vi "Pause.vi"(8 "error in (no error)":errorcluster, 11 "SS P100 Settings In":T1) -> (0 "error out":errorcluster, 1 "Connection Error":bool, 3 "SS P100 Settings Out":T1)   [LabVIEW 2018, in "Sonic Systems P100.lvlib"]
uses:
  Sonic Systems P100.lvlib
  Sonic Systems P100 Settings.ctl
  support/Support Library.lvlib
panel:
  out "read buffer":string
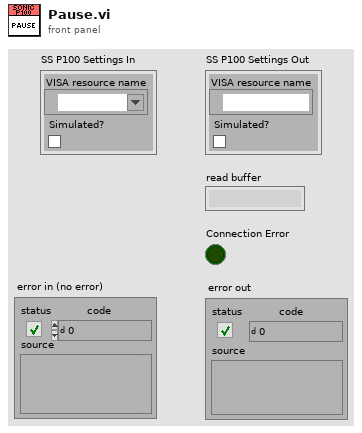
[diagram p1: front panel]
types:
  T1 = typedef "Sonic Systems P100.lvlib/Sonic Systems P100 Settings.ctl" = cluster{"VISA resource name":refnum<visa-resource-name>, "Simulated?":bool}
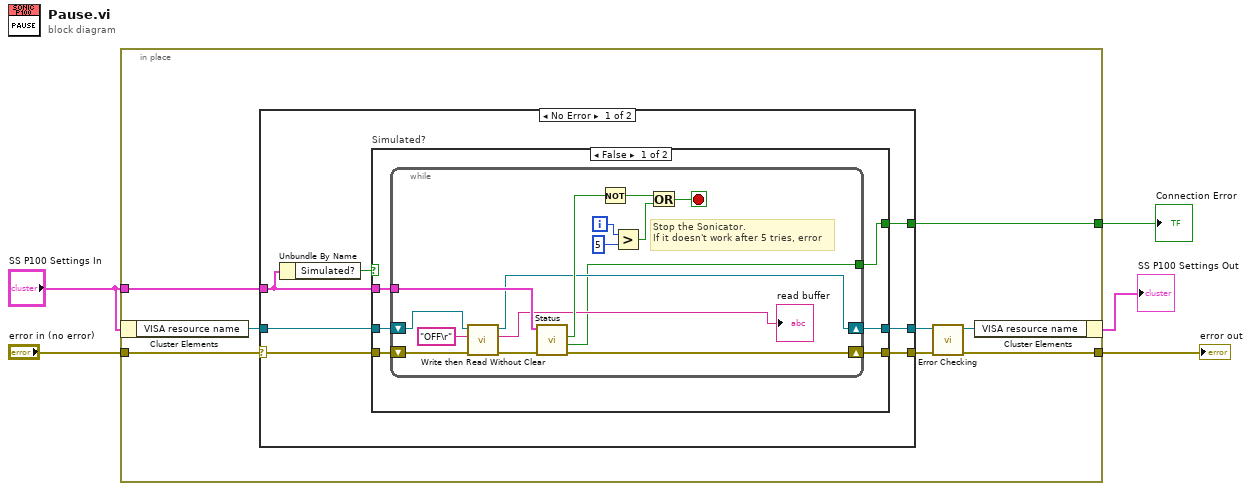
[diagram p0: block diagram]
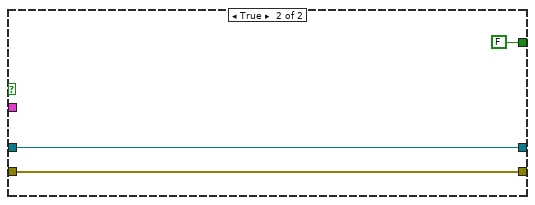
[diagram p2: hidden frame]
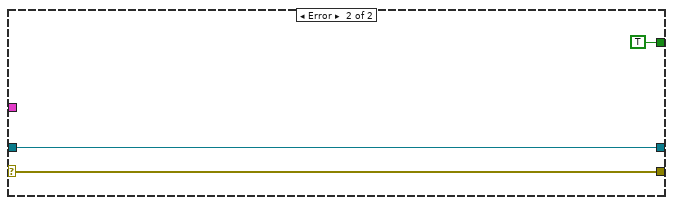
[diagram p3: hidden frame]
diagram:
  n1 = in-place {
    in-place-border: "error in (no error)" -> [w13]
    in-place-border: [w10] -> w4
    in-place-border: "SS P100 Settings In" -> [w9]
    in-place-border: [w6] -> w1
    n2 = in-place-cluster #1("SS P100 Settings In") -> ("VISA resource name"=w8:refnum<visa-resource-name>)
    n3 = case shown="No Error" w13 {
      selector: w13 -> [w20 w47]
      tunnel: w9 -> [w16 _]
      tunnel: [w19 w47] -> w11
      tunnel: [w18 w46] -> w12
      tunnel: w8 -> [w15 w46]
      tunnel: [w14 TRUE ("Connection Error")] -> w6
      frame No Error {
        n4 = Unbundle By Name(w16) -> ("Simulated?"=w17:bool)
        n5 = case "Simulated?" shown="False" w17 {
          tunnel: w20 -> [w24 w44]
          tunnel: [w22 w44] -> w19
          tunnel: [w26 w43] -> w18
          tunnel: w15 -> [w25 w43]
          tunnel: w16 -> [w23 _]
          tunnel: [w21 FALSE ("Connection Error")] -> w14
          frame False {
            n6 = while {
              tunnel: w23 -> [w41]
              shift-right: [w29] -> w26
              shift-left: w25 -> [w33]
              shift-right: [w40] -> w22
              shift-left: w24 -> [w31]
              tunnel: [w27] -> w21
              i -> [w38]
              stop <- w39 stop-if-true
              # "Stop the Sonicator. \nIf it doesn't work after 5 tries, error"
              n7 = call "Write then Read Without Clear.vi"("error in"=w31, "write buffer"="OFF\r" ("string"), "VISA resource name in"=w33) -> ("error out"=w30:errorcluster, "read buffer"=→"read buffer":string, "VISA resource name out"=w29:refnum<visa-resource-name>)  [unwired: 5 in, 1 out]
              n8 = call "Status.vi"("error in (no error)"=w30, "SS P100 Settings In"=w41) -> ("error out"=w40:errorcluster, "Connection Error"=w27:bool, "Running"=w34:bool)  [unwired: 4 in, 3 out]
              n9 = Not(x=w34) -> (.not. x?=w35:bool)
              n10 = Greater?(x=w38, y=5) -> (0:w36:bool)
              n11 = Or(x=w35, y=w36) -> (x .or. y?=w39:bool)
            }
          }
          frame True {
          }
        }
      }
      frame Error {
      }
    }
    n12 = call "Error Checking.vi"("error in (no error)"=w11, "VISA resource name"=w12) -> ("error out"=w10:errorcluster, "VISA resource name"=w7:refnum<visa-resource-name>)  [unwired: 7 in, 1 out]
    n13 = in-place-cluster #1("VISA resource name"=w7) -> (→"SS P100 Settings Out":T1)
  }
  "error out" <- w4
  "Connection Error" <- w1
